vi "ROI group-Save Load Groups setup.vi"(8 "error in (no error)":errorcluster, 9 "Function":T3=enum."Load file", 10 "Groups setup to save":T1[](array[typedef]) {"Group region specifier cluster"."Contours"."Type" items=["No Selection", "Point", "Line", "Rectangle", "Oval", "Polygon", "Freehand Region", "Annulus", "Unused2", "Unused3", "Broken Line", "Freehand Line", "Rotated Rectangle"]}, 11 "Complete overwrite (F)":bool) -> (0 "error out":errorcluster, 2 "Loaded groups setup":T1[](array[typedef]) {"Group region specifier cluster"."Contours"."Type" items=["No Selection", "Point", "Line", "Rectangle", "Oval", "Polygon", "Freehand Region", "Annulus", "Unused2", "Unused3", "Broken Line", "Freehand Line", "Rotated Rectangle"]})   [LabVIEW 2013]
uses:
  ROI Selection Interface/ROI group info cluster.ctl
  Experiment header interface/Typedefs/Save-Load-Save as-Load last enum.ctl
  Typedefs/Get-Set-Clear Control.ctl
  Global variables/gl_Functional Imaging-Global variables.vi
  <vilib>/Utility/xml.llb/Read From XML File(string).vi
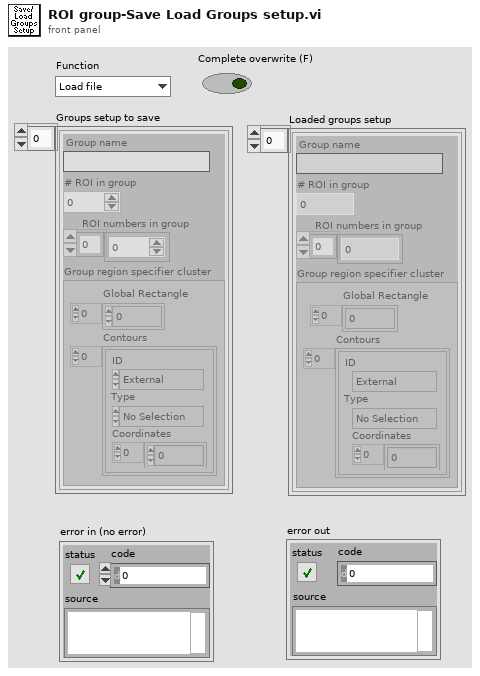
[diagram p1: front panel]
types:
  T1 = typedef "ROI group info cluster.ctl" = cluster{"Group name":string, "# ROI in group":i32, "ROI numbers in group":i32[], "Group region specifier cluster":T2}
  T2 = typedef "ROI Descriptor" = cluster{"Global Rectangle":i32[], "Contours":cluster{"ID":enum32{"External", "Internal"}, "Type":u32, "Coordinates":i32[]}[]}
  T3 = typedef "Save-Load-Save as-Load last enum.ctl" = enum16{"Save file", "Save file as", "Load file", "Load last file"}
  T4 = typedef "Get-Set-Clear Control.ctl" = enum16{"Get", "Set", "Clear"}
  T5 = typedef "Functional Imging UI Refs.ctl" = cluster{"Menu ref":refnum<k9>, "Image control":refnum<vi>, "VI ref":refnum<vi>, "XGrapher":refnum<vi>, "Smoothing":refnum<vi>, "POI Averaging":refnum<vi>, "Normalize":refnum<vi>, "POI data points in each trial":refnum<vi>, "Channel":refnum<vi>, "Experiment data folder path":refnum<vi>, "[ROI vis]":refnum<vi>, "[Groups] visbl":T6, "Group Name":refnum<vi>, "POI index":refnum<vi>, "Trial No.":refnum<vi>, "Intensity Zoom":refnum<vi>, "Trial Cursor Enabled":refnum<vi>, "Number of Trials (ind 1)":refnum<vi>, "Number of Trials (ind 2)":refnum<vi>, "MiniScans Available":refnum<vi>, "POI Available":refnum<vi>, "Defer graph updates":refnum<vi>, "Waveform selector":refnum<vi>, "#of selected POI":refnum<vi>, "#of selected MiniScans":refnum<vi>, "#of selected groups":refnum<vi>, "Max Z-Projection":refnum<vi>, "Z-Plane Selector":refnum<vi>, "Index of miniscan point to visualise":refnum<vi>, "ROI vis. mode":refnum<vi>, "Total # of points":refnum<vi>, "Index of group clicked on":refnum<vi>, "Pane 1":refnum<vi>, "Pane 2":refnum<vi>, "Pane 3":refnum<vi>, "Pane 4":refnum<vi>, "Pane 5":refnum<vi>, "Pane 6":refnum<vi>, "Deselect all ROI":refnum<vi>, "Deselect all groups":refnum<vi>}
  T6 = typedef "Groups array referecne.ctl" = refnum<vi>
  T7 = typedef "Fixed strings.ctl" = cluster{"ROI file name":string, "Normalised ROI file name":string, "Zplane Pockels values file name":string, "Functional data folder name":string, "Experiment Header file name":string, "Z-stack images folder name":string, "Groups setup rel. path":string, "Groups text file rel. path":string, "TDMS files folder name (F.img)":string, "TDMS files folder name (V.acq)":string, "TDMS files folder name (Pl.acq)":string, "Cycle rel times sequence file":string, "Dynamically called VIs folder name":string, "Time Series folder base name":string}
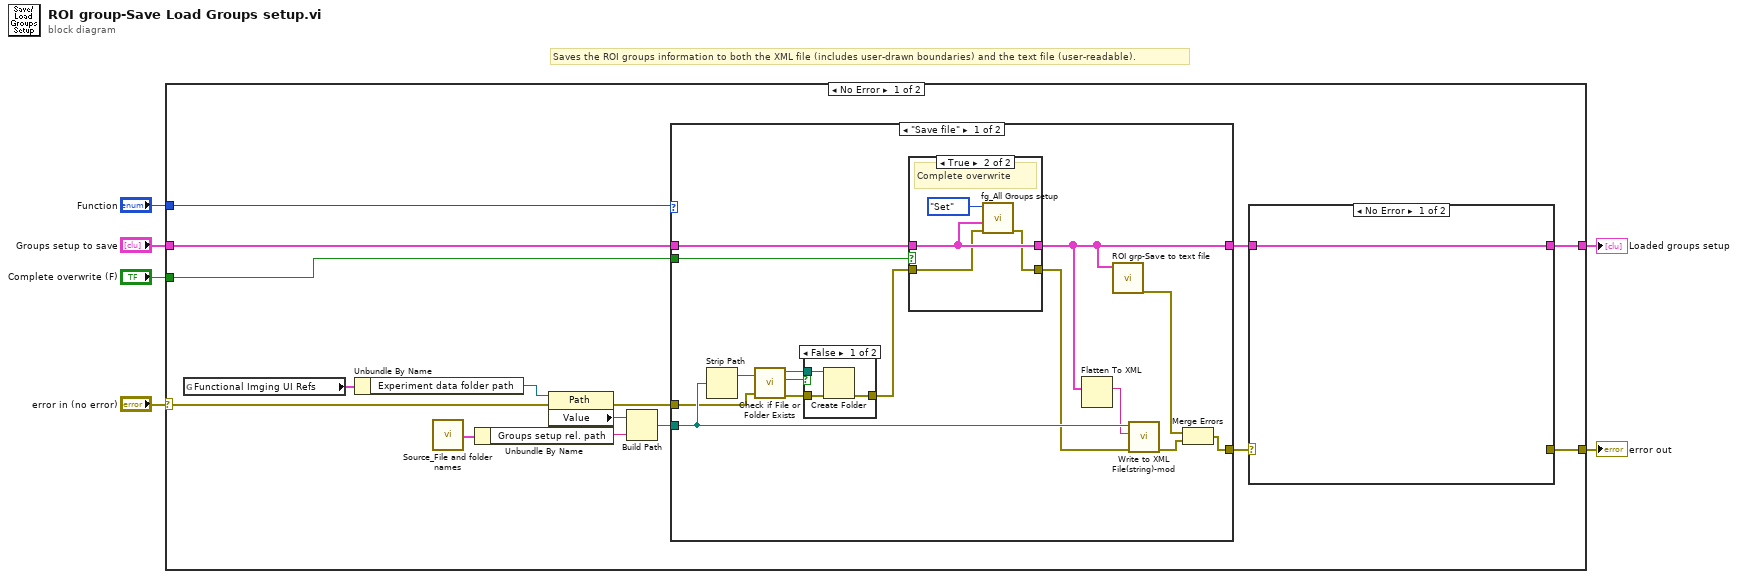
[diagram p0: block diagram]
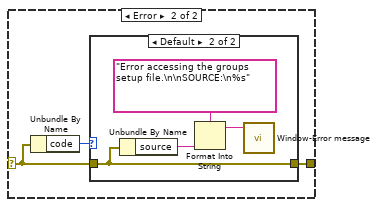
[diagram p2: hidden frame]
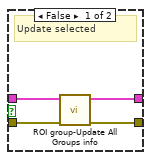
[diagram p4: hidden frame]
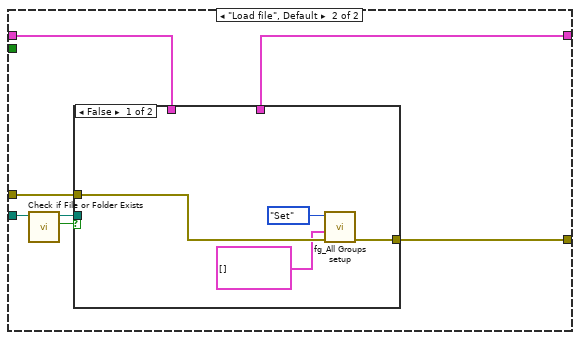
[diagram p6: hidden frame]
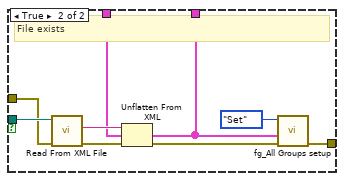
[diagram p7: hidden frame]
diagram:
  # "Saves the ROI groups information to both the XML file (includes user-drawn boundaries) and the text file (user-readable)."
  n1 = case shown="No Error" "error in (no error)" {
    selector: "error in (no error)" -> [w14 w77]
    tunnel: "Groups setup to save" -> [w18 _]
    tunnel: "Function" -> [w17 _]
    tunnel: [w10 _] -> w4
    tunnel: [w15 w77] -> w3
    tunnel: "Complete overwrite (F)" -> [w7 _]
    frame No Error {
      n2 = global read "gl_Functional Imaging-Global variables.vi" "Functional Imging UI Refs"() -> (w9:T5)
      n3 = Unbundle By Name(w9) -> ("Experiment data folder path"=w8:refnum<vi>)
      n4 = call "Source_File and folder names.vi"() -> ("Fixed strings"=w21:T7)  [unwired: 1 in]
      n5 = Unbundle By Name(w21) -> ("Groups setup rel. path"=w20:string)
      n6 = property on="Property Node" class="Path"(reference=w8, error in=w14) -> (error out=w12:errorcluster, "Value"=w19:path)  [unwired: 1 out]
      n7 = Build Path(base path=w19, name or relative path=w20) -> (appended path=w13:path)
      n8 = case shown="\"Save file\"" w17 {
        tunnel: [w32 w60] -> w16
        tunnel: w13 -> [w42 w59]
        tunnel: w18 -> [w38 w63]
        tunnel: [w34 w61] -> w11
        tunnel: w12 -> [w40 w62]
        tunnel: w7 -> [w30 _]
        frame "Save file" {
          n9 = Strip Path(path=w42) -> (stripped path=w41:path)  [unwired: 1 out]
          n10 = call <vilib>:"Check if File or Folder Exists.vi"("error in (no error)"=w40, "path"=w41) -> ("error out"=w43:errorcluster, "file or folder exists?"=w39:bool, "dup path"=w44:path)  [unwired: 7 in]
          n11 = case shown="False" w39 {
            tunnel: w44 -> [w55 _]
            tunnel: w43 -> [w54 w56]
            tunnel: [w53 w56] -> w36
            frame False {
              n12 = Create Folder(path (use dialog)=w55, error in=w54) -> (error out=w53:errorcluster)  [unwired: 1 in, 2 out]
            }
            frame True {
            }
          }
          n13 = case shown="True" w30 {
            tunnel: w38 -> [w48 w51]
            tunnel: w36 -> [w47 w49]
            tunnel: [w46 w50] -> w35
            tunnel: [w45 w51] -> w34
            frame False {
              # "Update selected"
              n14 = call "ROI group-Update All Groups info.vi"("error in (no error)"=w47, "Groups setup to add/update"=w48) -> ("error out"=w46:errorcluster, "Updated \"All groups\" setup"=w45:T1[])  [unwired: 8 in]
            }
            frame True {
              # "Complete overwrite"
              n15 = call "fg_All Groups setup.vi"("error in (no error)"=w49, "Groups setup in"=w51, "Function"=Get-Set-Clear_Control."Set") -> ("error out"=w50:errorcluster)  [unwired: 7 in, 1 out]
            }
          }
          n16 = Flatten To XML(anything=w34) -> (xml string=w37:string)
          n17 = call "ROI grp-Save to text file.vi"("Groups setup to add/update"=w34) -> ("error out"=w31:errorcluster)  [unwired: 10 in]
          n18 = call "Write to XML File(string)-mod.vi"("error in (no error)"=w35, "XML Input"=w37, "XML File Path"=w42) -> ("error out"=w33:errorcluster)  [unwired: 6 in, 2 out]
          n19 = Merge Errors(w31, w33) -> (w32:errorcluster)
        }
        frame "Load file", Default {
          n20 = call <vilib>:"Check if File or Folder Exists.vi"("path"=w59) -> ("file or folder exists?"=w57:bool, "dup path"=w58:path)  [unwired: 8 in, 1 out]
          n21 = case shown="False" w57 {
            tunnel: w63 -> [_ w75]
            tunnel: w58 -> [_ w74]
            tunnel: w62 -> [w66 w72]
            tunnel: [_ w70] -> w61
            tunnel: [w65 w68] -> w60
            frame False {
              n22 = call "fg_All Groups setup.vi"("error in (no error)"=w66, "Groups setup in"=T1[] [], "Function"=Get-Set-Clear_Control."Set") -> ("error out"=w65:errorcluster)  [unwired: 7 in, 1 out]
            }
            frame True {
              # "File exists"
              n23 = call-poly <vilib>:"Read From XML File.vi"("error in (no error)"=w72, "XML File Path"=w74) -> ("error out"=w73:errorcluster, "XML Elements"=w76:string)  [unwired: 7 in, 1 out]
              n24 = Unflatten From XML(xml string=w76, type=w75, error in (no error)=w73) -> (value=w70:T1[], error out=w69:errorcluster)
              n25 = call "fg_All Groups setup.vi"("error in (no error)"=w69, "Groups setup in"=w70, "Function"=Get-Set-Clear_Control."Set") -> ("error out"=w68:errorcluster)  [unwired: 7 in, 1 out]
            }
          }
        }
      }
      n26 = case shown="No Error" w16 {
        selector: w16 -> [_ w23]
        tunnel: [_ w24] -> w15
        tunnel: w11 -> [w22 _]
        tunnel: [w22 _] -> w10
        frame No Error {
        }
        frame Error {
          n27 = Unbundle By Name(w23) -> ("code"=w25:i32)
          n28 = case shown="Default" w25 {
            tunnel: w23 -> [_ w26]
            tunnel: [_ w26] -> w24
            frame 7 {
              # "Clears error 7 when a groups setup file does not already exist."
            }
            frame Default {
              n29 = Unbundle By Name(w26) -> ("source"=w28:string)
              n30 = Format Into String(format string="Error accessing the groups setup file.\n\nSOURCE:\n%s", w28) -> (resulting string=w27:string)  [unwired: 2 in, 1 out]
              n31 = call "Window-Error message.vi"("Message"=w27) -> ()  [unwired: 10 in, 1 out]
            }
          }
        }
      }
    }
    frame Error {
    }
  }
  "error out" <- w3
  "Loaded groups setup" <- w4
